vi "reverse_remainder_WIP.vi"() -> ()   [LabVIEW 2019]
panel:
  out "R":i32[](array[numeric])
  out "R 5":dbl
  out "R 4":dbl
  out "R 3":dbl
  out "R 2":dbl
  in  "m":i32
  in  "N":i32
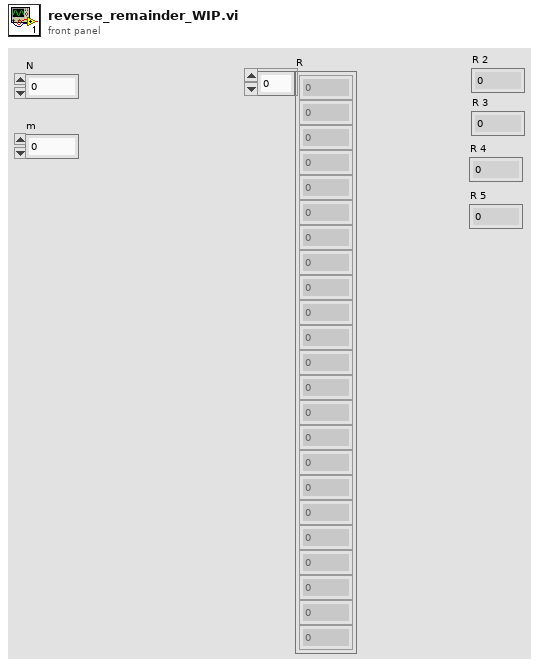
[diagram p1: front panel]
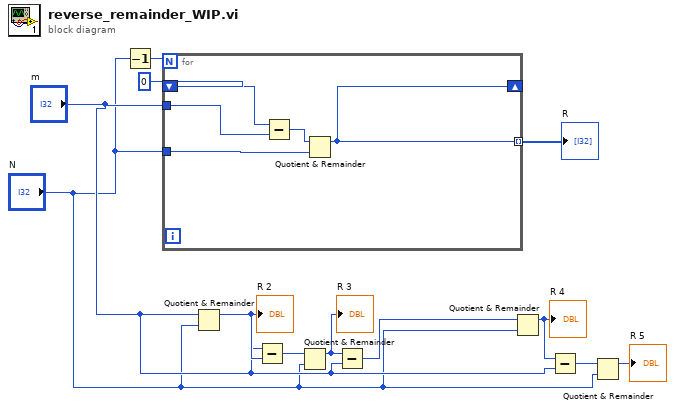
[diagram p0: block diagram]
diagram:
  n1 = Decrement(x="N") -> (x-1=w3:i32)
  n2 = for {
    N: w3 -> [_]
    shift-right: [w13] -> _
    shift-left: 0 -> [w16]
    tunnel: "m" -> [w15]
    tunnel: "N" -> [w14]
    tunnel: [w13] -> w4 mode=indexing
    n3 = Subtract(x=w16, y=w15) -> (x-y=w17:i32)
    n4 = Quotient & Remainder(x=w17, y=w14) -> (x-y*floor(x/y)=w13:i32)  [unwired: 1 out]
  }
  "R" <- w4
  n5 = Quotient & Remainder(x="m", y="N") -> (x-y*floor(x/y)=w11:i32)  [unwired: 1 out]
  "R 2" <- w11
  n6 = Subtract(x="m", y=w11) -> (x-y=w10:i32)
  n7 = Quotient & Remainder(x=w10, y="N") -> (x-y*floor(x/y)=w8:i32)  [unwired: 1 out]
  "R 3" <- w8
  n8 = Subtract(x=w8, y="m") -> (x-y=w9:i32)
  n9 = Quotient & Remainder(x=w9, y="N") -> (x-y*floor(x/y)=w7:i32)  [unwired: 1 out]
  "R 4" <- w7
  n10 = Subtract(x=w7, y="m") -> (x-y=w6:i32)
  n11 = Quotient & Remainder(x=w6, y="N") -> (x-y*floor(x/y)=→"R 5":i32)  [unwired: 1 out]
